vi "CPP_Aeroprobe_TimeSeries-AeroFlow.vi"() -> (5 "Plug in titles":string[](array[string]), 7 "Plug in values":string[](array[string]))   [LabVIEW 2013]
uses:
  Globals/Meas_global.vi
panel:
  out "AvgReduction (ms)":dbl
  out "reduction ms":u32
  in  "Calibration Folder Path":path=path "M:/Preferences/Rig_Setups/All_Rigs/Calibrations/5HoleProbe"
  in  "Correction File Path":path=path "M:/Preferences/Rig_Setups/All_Rigs/TubingCompensation/5HPTubingCorrection12066.xls"
  in  "Apply Phase Correction?":bool=TRUE
  out "DataArray":dbl[](array[numeric])
  out "Zeroes":dbl[](array[numeric])
  # "!! 5-hole 1-5 must be connected to Channels 1-5 !!"
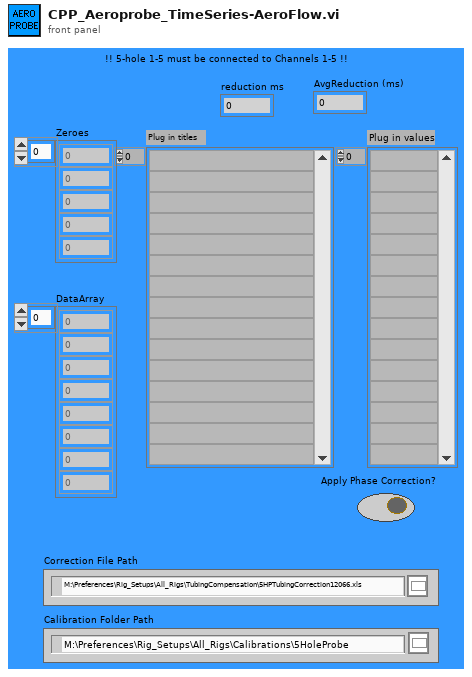
[diagram p1: front panel]
types:
  T1 = typedef "Analysis_info_cluster.ctl" = cluster{"Colour":u32, "Inst type":T2, "Inst name":string, "Symbol":string, "Code name":string, "Extra Info":string, "Inst Array":T3, "Extra Titles":string[], "Extra Values":string[], "U":dbl, "u^2":dbl, "u^3":dbl, "u^4":dbl, "Skew_u":dbl, "Kurt_u":dbl, "Sd Error in Mean":dbl, "% u'/U":dbl, "X":dbl, "Y":dbl, "Z":dbl, "Timescale integral to 25%":dbl, "Sd Error in Variance":dbl, "Calib File":path, "Calib Constants":dbl[], "Output Position":bool, "Full Stats":bool, "Av Sampling Rate":dbl, "Av No of Samples":dbl, "Total Meas Time (s)":dbl, "ADAM Ch Name":string}
  T2 = typedef "Inst_type.ctl" = enum16{"Propeller anemometer", "Raw voltage", "Pressure Transducer", "Pitot-static tube", "Preston tube", "Hot wire", "Cross wire 1", "Cross wire 2", "Generic Linear", "Generic Polynomial", "Generic BackPoly", "Fast FID", "Thermocouple", "Cold wire", "Pulsed Wire", "LDA Vel", "LDA Tran time", "LDA Arr time"}
  T3 = typedef "Instrument_Array.ctl" = enum16{"PWA", "LDA", "Analogue"}
  T4 = cluster{"Analysis Info cluster[0]":T1, "Analysis Info cluster[1]":T1, "Analysis Info cluster[2]":T1, "Analysis Info cluster[3]":T1, "Analysis Info cluster[4]":T1, "Analysis Info cluster[5]":T1, "Analysis Info cluster[6]":T1}
  T5 = typedef "Time_Trace_Cluster.ctl" = cluster{"Weighting":dbl[], "Time (s)":dbl[], "Voltage":dbl[], "Eng Values":dbl[]}
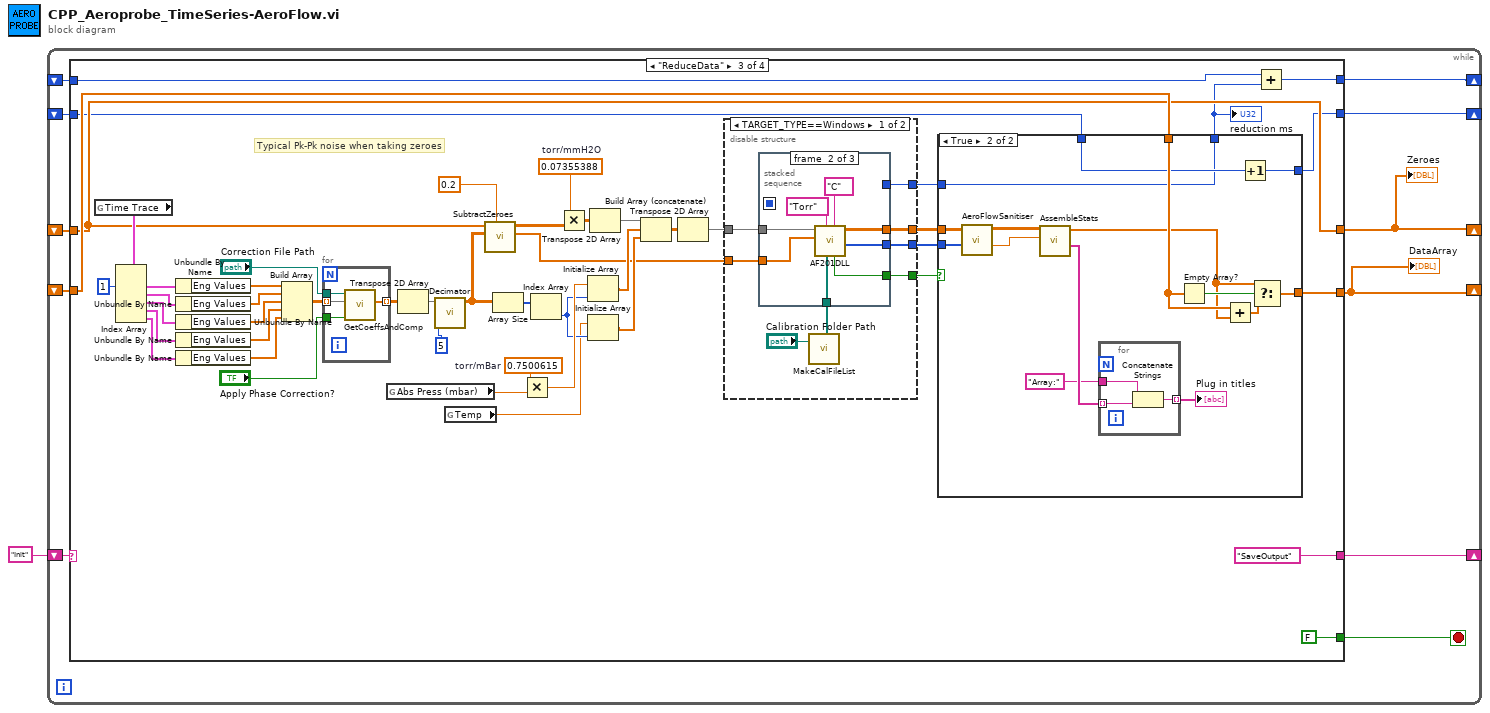
[diagram p0: block diagram]
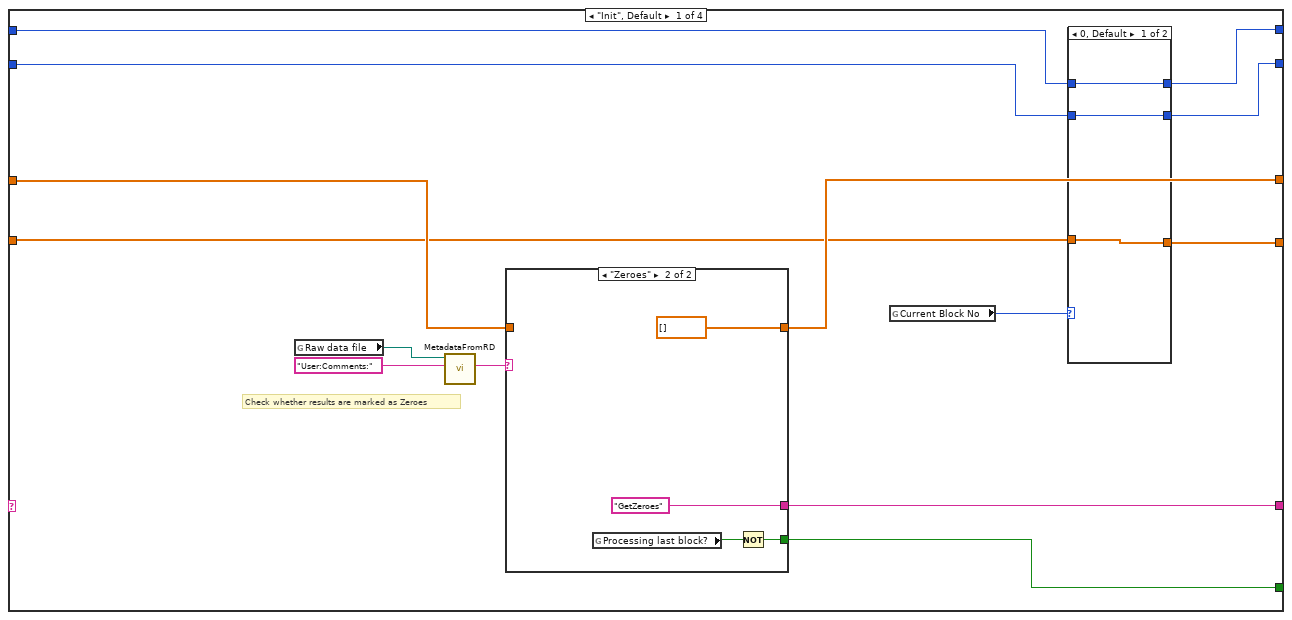
[diagram p2: hidden frame]
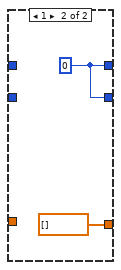
[diagram p3: hidden frame]
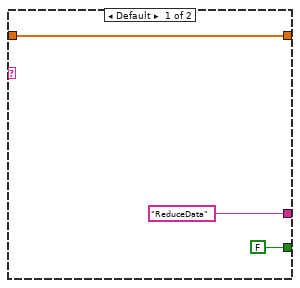
[diagram p4: hidden frame]
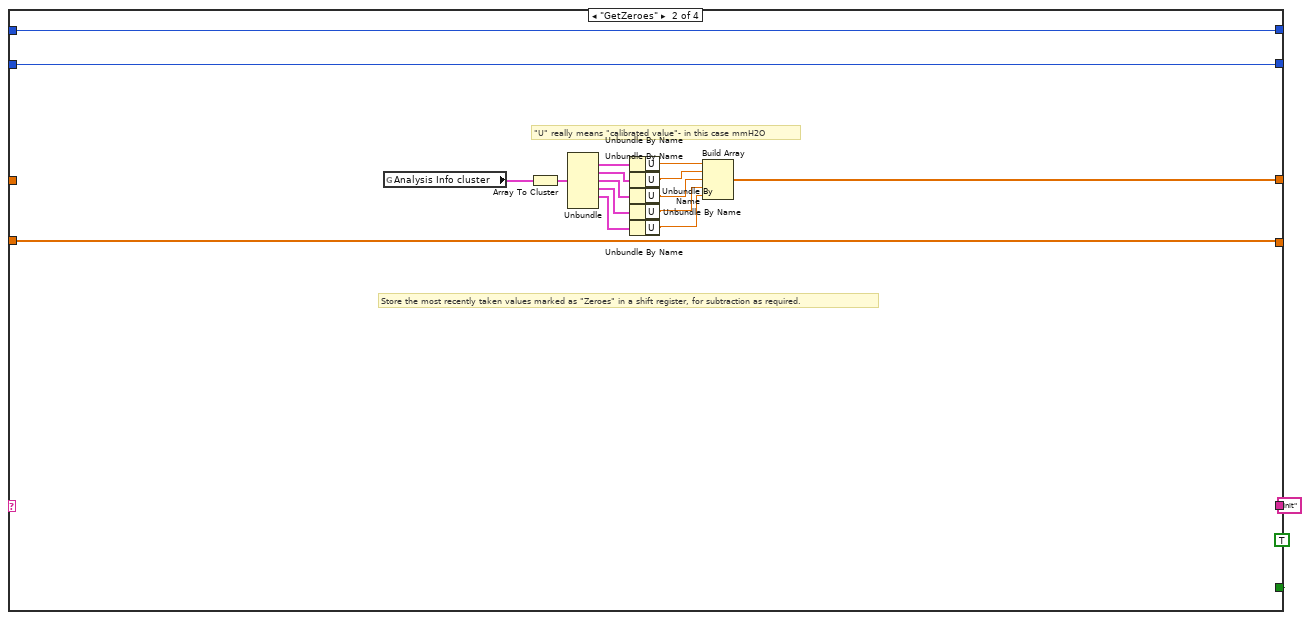
[diagram p5: hidden frame]
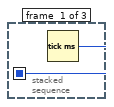
[diagram p6: hidden frame]
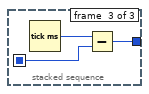
[diagram p7: hidden frame]
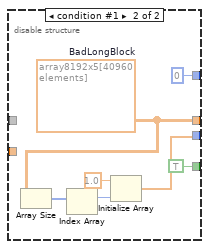
[diagram p8: hidden frame]
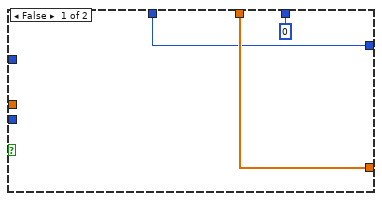
[diagram p9: hidden frame]
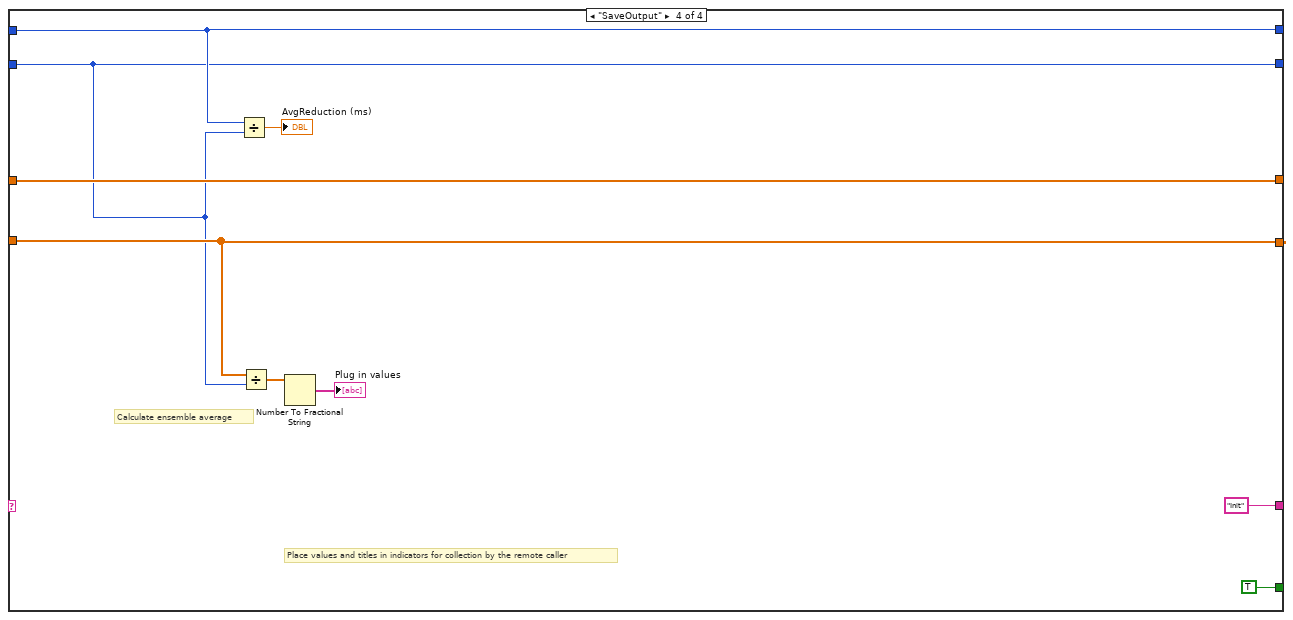
[diagram p10: hidden frame]
diagram:
  n1 = while {
    shift-right: [w11] -> _
    shift-left: "Init" -> [w12]
    shift-right: [w10] -> _
    shift-left: _ -> [w9]
    shift-right: [w8] -> _
    shift-left: _ -> [w7]
    shift-right: [w5] -> _
    shift-left: _ -> [w4]
    shift-right: [w2] -> _
    shift-left: _ -> [w3]
    stop <- w6 stop-if-true
    n2 = case shown="\"ReduceData\"" w12 {
      tunnel: [w26 "Init" "SaveOutput" "Init"] -> w11
      tunnel: [w20 w43 w81 w166] -> w10
      tunnel: w9 -> [w21 _ w81 w166]
      tunnel: [w18 w41 w90 w162] -> w8
      tunnel: w7 -> [w17 w41 w91 w162]
      tunnel: [w22 TRUE FALSE TRUE] -> w6
      tunnel: [w16 w40 w67 w160] -> w5
      tunnel: w4 -> [w14 w40 w65 w160]
      tunnel: w3 -> [w13 w39 w61 w158]
      tunnel: [w15 w39 w60 w158] -> w2
      frame "Init", Default {
        # "Check whether results are marked as Zeroes"
        n3 = global read "Meas_global.vi" "Raw data file"() -> (w25:path)
        n4 = call "MetadataFromRD.vi"("ChannelName"="User:Comments:", "Raw data file"=w25) -> ("ValueString"=w23:string)  [unwired: 8 in, 1 out]
        n5 = case shown="\"Zeroes\"" w23 {
          tunnel: ["ReduceData" "GetZeroes"] -> w26
          tunnel: [FALSE w37] -> w22
          tunnel: w21 -> [w32 _]
          tunnel: [w32 dbl[] [] ("t")] -> w20
          frame Default {
          }
          frame "Zeroes" {
            n6 = global read "Meas_global.vi" "Processing last block?"() -> (w36:bool)
            n7 = Not(x=w36) -> (.not. x?=w37:bool)
          }
        }
        n8 = global read "Meas_global.vi" "Current Block No"() -> (w19:i32)
        n9 = case shown="0, Default" w19 {
          tunnel: [w29 dbl[] [] ("t")] -> w18
          tunnel: w17 -> [w29 _]
          tunnel: [w28 w30] -> w16
          tunnel: [w27 w30] -> w15
          tunnel: w14 -> [w28 _]
          tunnel: w13 -> [w27 _]
          frame 0, Default {
          }
          frame 1 {
            w30 = u32 0
          }
        }
      }
      frame "GetZeroes" {
        # "Store the most recently taken values marked as \"Zeroes\" in a shift register, for subtraction as required."
        # "\"U\" really means \"calibrated value\"- in this case mmH2O"
        n10 = global read "Meas_global.vi" "Analysis Info cluster"() -> (w45:T1[])
        n11 = Array To Cluster(array=w45) -> (cluster=w51:T4)
        n12 = Unbundle(w51) -> ("Analysis Info cluster[1]"=w52:T1, "Analysis Info cluster[2]"=w53:T1, "Analysis Info cluster[3]"=w54:T1, "Analysis Info cluster[4]"=w55:T1, "Analysis Info cluster[5]"=w56:T1)  [unwired: 2 out]
        n13 = Unbundle By Name(w52) -> ("U"=w50:dbl)
        n14 = Unbundle By Name(w53) -> ("U"=w49:dbl)
        n15 = Unbundle By Name(w54) -> ("U"=w48:dbl)
        n16 = Unbundle By Name(w55) -> ("U"=w47:dbl)
        n17 = Unbundle By Name(w56) -> ("U"=w46:dbl)
        n18 = Build Array(w50, w49, w48, w47, w46) -> (w43:dbl[])
      }
      frame "ReduceData" {
        w83 = 0.07355388  # torr/mmH2O
        w84 = 0.7500615  # torr/mBar
        # "Typical Pk-Pk noise when taking zeroes"
        n19 = global read "Meas_global.vi" "Time Trace"() -> (w95:T5[])
        n20 = Index Array(array=w95, index #1=1 ("index")) -> (element #1=w94:T5, element #2=w103:T5, element #3=w102:T5, element #4=w101:T5, element #5=w100:T5)  [unwired: 4 in]
        n21 = Unbundle By Name(w94) -> ("Eng Values"=w93:dbl[])
        n22 = Unbundle By Name(w103) -> ("Eng Values"=w99:dbl[])
        n23 = Unbundle By Name(w102) -> ("Eng Values"=w98:dbl[])
        n24 = Unbundle By Name(w101) -> ("Eng Values"=w97:dbl[])
        n25 = Unbundle By Name(w100) -> ("Eng Values"=w96:dbl[])
        n26 = Build Array(w93, w99, w98, w97, w96) -> (w89:dbl[][])
        n27 = for {
          tunnel: w89 -> [w157] mode=indexing
          tunnel: [w156] -> w86 mode=indexing
          tunnel: "Apply Phase Correction?" -> [w155]
          tunnel: "Correction File Path" -> [w154]
          n28 = call "GetCoeffsAndComp.vi"("Apply Phase Correction?"=w155, "mutedData"=w157, "TubingCorrectionFile (pre-set!)"=w154) -> ("boostedData"=w156:dbl[])  [unwired: 8 in]
        }
        n29 = global read "Meas_global.vi" "Abs Press (mbar)"() -> (w85:dbl)
        n30 = Transpose 2D Array(2D array=w86) -> (transposed array=w69:dbl[][])
        n31 = call "Decimator.vi"("Divider"=5, "Array In"=w69) -> ("Array Out"=w68:dbl[][])  [unwired: 9 in]
        n32 = global read "Meas_global.vi" "Temp"() -> (w71:dbl)
        n33 = call "SubtractZeroes.vi"("NoiseFloorValue (Pressure Units)"=0.2, "RawPressure"=w68, "Zeroes"=w81) -> ("MaxdP"=w57:dbl[], "ZeroedPressure"=w82:dbl[][])  [unwired: 6 in, 1 out]
        n34 = Array Size(array=w68) -> (size(s)=w80:i32[])
        n35 = Multiply(x=w84, y=w85) -> (x*y=w79:dbl)
        n36 = Index Array(array=w80) -> (element=w78:i32)  [unwired: 1 in]
        n37 = Multiply(x=w83, y=w82) -> (x*y=w77:dbl[][])
        n38 = Initialize Array(w79, w78) -> (w75:dbl[])
        n39 = Initialize Array(w71, w78) -> (w74:dbl[])
        n40 = Transpose 2D Array(2D array=w77) -> (transposed array=w73:dbl[][])
        n41 = Build Array (concatenate)(w73, w75, w74) -> (w76:dbl[][])
        n42 = Transpose 2D Array(2D array=w76) -> (transposed array=w72:dbl[][])
        n43 = disable-structure shown="TARGET_TYPE==Windows" {
          disable-tunnel: w72 -> [w111 _]
          disable-tunnel: [w110 u32 0] -> w64
          disable-tunnel: [w109 w130] -> w63
          disable-tunnel: [w108 TRUE ("GoodBlock")] -> w62
          disable-tunnel: [w107 w127] -> w59
          disable-tunnel: w57 -> [w106 _]
          frame condition #0 (active) {
            n44 = call "MakeCalFileList.vi"("Calibration Folder Path"="Calibration Folder Path") -> ("Calibration File(s)"=w112:path[])  [unwired: 1 in, 1 out]
            n45 = stacked-sequence {
              seq-local: [w114 _ _] -> [_ _ w125]
              tunnel: w111 -> [_ w122 _]
              tunnel: w112 -> [_ w115 _]
              tunnel: [_ _ w124] -> w110
              tunnel: [_ w119 _] -> w109
              tunnel: [_ w118 _] -> w108
              tunnel: [_ w117 _] -> w107
              tunnel: w106 -> [_ w116 _]
              frame #0 {
                n46 = Tick Count (ms)() -> (millisecond timer value=w114:u32)
              }
              frame #1 {
                n47 = call "AF201DLL.vi"("Temperature Units"="C", "Calibration File(s)"=w115, "Pressure Units"="Torr", "MaxdP(mmH2O)"=w116, "Data to Reduce"=w122) -> ("Error_Flags"=w117:i32[], "VmagUVWCone"=w119:dbl[][], "GoodBlock"=w118:bool)  [unwired: 4 in]
              }
              frame #2 {
                n48 = Tick Count (ms)() -> (millisecond timer value=w123:u32)
                n49 = Subtract(x=w123, y=w125) -> (x-y=w124:u32)
              }
            }
          }
          frame condition #1 {
            w130 = dbl[][] array8192x5[40960 elements]  # BadLongBlock
            n50 = Array Size(array=w130) -> (size(s)=w129:i32[])
            n51 = Index Array(array=w129) -> (element=w128:i32)  [unwired: 1 in]
            n52 = Initialize Array(1.0 ("element"), w128) -> (w127:dbl[])
          }
        }
        n53 = case shown="True" w62 {
          tunnel: w91 -> [w135 w150]
          tunnel: [w135 w147] -> w90
          tunnel: [u32 0 w136] -> w66
          tunnel: w64 -> [_ w136]
          tunnel: w63 -> [_ w140]
          tunnel: w61 -> [w133 w145]
          tunnel: [w133 w144] -> w60
          tunnel: w59 -> [_ w137]
          frame False {
          }
          frame True {
            n54 = call "AeroFlowSanitiser.vi"("Error_Flags"=w137, "VmagUVWConeDirty"=w140) -> ("GoodFraction"=w138:dbl, "VmagUVWConeClean"=w139:dbl[][])  [unwired: 8 in]
            n55 = call "AssembleStats.vi"("ValidFraction"=w138, "VmagUVWCone"=w139) -> ("Plug in titles"=w143:string[], "StatsArray"=w146:dbl[])  [unwired: 8 in]
            n56 = for {
              tunnel: w143 -> [w153] mode=indexing
              tunnel: "Array:" -> [w152]
              tunnel: [w151] -> w141 mode=indexing
              n57 = Concatenate Strings(w152, w153) -> (w151:string)
            }
            "Plug in titles" <- w141
            n58 = Empty Array?(array=w150) -> (empty?=w149:bool)
            n59 = Add(x=w150, y=w146) -> (x+y=w148:dbl[])
            n60 = Increment(x=w145) -> (x+1=w144:u32)
            n61 = Select(t=w146, s=w149, f=w148) -> (s? t:f=w147:dbl[])
          }
        }
        "reduction ms" <- w66
        n62 = Add(x=w65, y=w66) -> (x+y=w67:u32)
      }
      frame "SaveOutput" {
        # "Place values and titles in indicators for collection by the remote caller"
        # "Calculate ensemble average"
        n63 = Divide(x=w160, y=w158) -> (x/y=→"AvgReduction (ms)":dbl)
        n64 = Divide(x=w162, y=w158) -> (x/y=w161:dbl[])
        n65 = Number To Fractional String(number=w161) -> (F-format string=→"Plug in values":string[])  [unwired: 3 in]
      }
    }
    "Zeroes" <- w10
    "DataArray" <- w8
  }
